vi "Set Remote Terminal Name.vi"(8 "error in":errorcluster, 10 "terminal name":string, 11 "remote terminal":T1 format="%.0x") -> (0 "error out":errorcluster, 3 "remote terminal out":T1 format="%.0x")   [LabVIEW 2020, in "AIM MIL-STD-1553 Scripting.lvlib"]
doc: "Sets <b>name</b> for the specified <b>remote terminal</b>."
uses:
  AIM MIL-STD-1553 Scripting.lvlib
  <vilib>/NI VeriStand/Custom Device API/Custom Device Item Ref.ctl
  <vilib>/NI VeriStand/Custom Device API/Custom Device API.lvlib
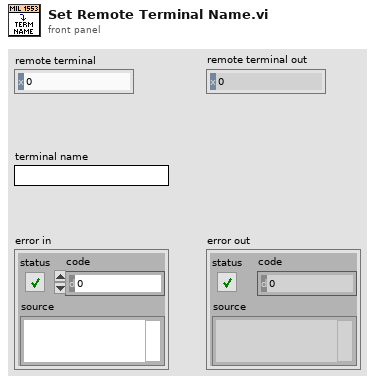
[diagram p1: front panel]
types:
  T1 = typedef "Custom Device API.lvlib/Custom Device Item Ref.ctl" = u64
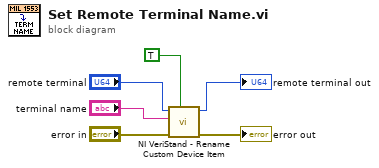
[diagram p0: block diagram]
diagram:
  n1 = call <vilib>:"NI VeriStand - Rename Custom Device Item.vi"("Force Rename (F)"=TRUE, "error in (no error)"="error in", "New Name"="terminal name", "Item Ref in"="remote terminal") -> ("error out"=→"error out":errorcluster, "Item Ref out"=→"remote terminal out":T1)  [unwired: 5 in, 1 out]
